vi "Get Absolute Position of SubVI.vi"(8 "Error In":errorcluster, 10 "SubVI Reference":refnum<vi>, 11 "VI Reference":refnum<vi>) -> (0 "Error Out":errorcluster, 3 "Position":cluster{i32, i32})   [LabVIEW 2019, in "Peek Window.lvlib"]
uses:
  Peek Window.lvlib
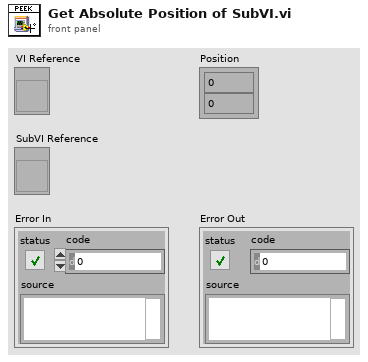
[diagram p1: front panel]
types:
  T1 = typedef "LVPointTypeDef.ctl" = cluster{"Horizontal":i16, "Vertical":i16}
  T2 = typedef "LVRectTypeDef.ctl" = cluster{"Left":i16, "Top":i16, "Right":i16, "Bottom":i16}
  T3 = typedef "LVPositionTypeDef.ctl" = cluster{"Left":i32, "Top":i32}
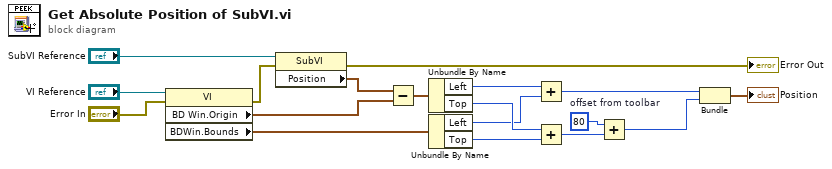
[diagram p0: block diagram]
diagram:
  w14 = 80  # offset from toolbar
  n1 = property class="VI"(reference="VI Reference", error in="Error In") -> (error out=w1:errorcluster, "BD Win.Origin"=w5:T1, "BDWin.Bounds"=w4:T2)  [unwired: 1 out]
  n2 = property class="SubVI"(reference="SubVI Reference", error in=w1) -> (error out=→"Error Out":errorcluster, "Position"=w6:T3)  [unwired: 1 out]
  n3 = Subtract(x=w6, y=w5) -> (x-y=w7:T3)
  n4 = Unbundle By Name(w7) -> ("Left"=w8:i32, "Top"=w10:i32)
  n5 = Unbundle By Name(w4) -> ("Left"=w9:i16, "Top"=w11:i16)
  n6 = Add(x=w8, y=w9) -> (x+y=w12:i32)
  n7 = Add(x=w10, y=w11) -> (x+y=w13:i32)
  n8 = Add(x=w14, y=w13) -> (x+y=w15:i32)
  n9 = Bundle(w12, w15) -> (→"Position":cluster{i32, i32})  [unwired: 1 in]
